vi "error_anal.vi"(9 "data":dbl[][](array[numeric])=array1024x498[509952 elements], 11 "wavelength":dbl[](array[numeric])=[350.0, 350.3, 350.6, 350.9, 351.2, 351.5, 351.8, 352.1, 352.4, 352.7, 353.0, 353.3, 353.6, 353.9, 354.2, 354.5, 354.8, 355.1, 355.4, 355.7, 356.0, 356.3, 356.6, 356.9, 357.2, 357.5, 357.8, 358.1, 358.4, 358.7, 359.0, 359.3, 359.6, 359.9, 360.2, 360.5, 360.8, 361.1, 361.4, 361.7, 362.0, 362.3, 362.6, 362.9, 363.2, 363.5, 363.8, 364.1, 364.4, 364.7, 365.0, 365.3, 365.6, 365.9, 366.2, 366.5, 366.8, 367.1, 367.4, 367.7, 368.0, 368.3, 368.6, 368.9, 369.2, 369.5, 369.8, 370.1, 370.4, 370.7, 371.0, 371.3, 371.6, 371.9, 372.2, 372.5, 372.8, 373.1, 373.4, 373.7, 374.0, 374.3, 374.6, 374.9, 375.2, 375.5, 375.8, 376.1, 376.4, 376.7, 377.0, 377.3, 377.6, 377.9, 378.2, 378.5, 378.8, 379.1, 379.4, 379.7, 380.0, 380.3, 380.6, 380.9, 381.2, 381.5, 381.8, 382.1, 382.4, 382.7, 383.0, 383.3, 383.6, 383.9, 384.2, 384.5, 384.8, 385.1, 385.4, 385.7, 386.0, 386.3, 386.6, 386.9, 387.2, 387.5, 387.8, 388.1, 388.4, 388.7, 389.0, 389.3, 389.6, 389.9, 390.2, 390.5, 390.8, 391.1, 391.4, 391.7, 392.0, 392.3, 392.6, 392.9, 393.2, 393.5, 393.8, 394.1, 394.4, 394.7, 395.0, 395.3, 395.6, 395.9, 396.2, 396.5, 396.8, 397.1, 397.4, 397.7, 398.0, 398.3, 398.6, 398.9, 399.2, 399.5, 399.8, 400.1, 400.4, 400.7, 401.0, 401.3, 401.6, 401.9, 402.2, 402.5, 402.8, 403.1, 403.4, 403.7, 404.0, 404.3, 404.6, 404.9, 405.2, 405.5, 405.8, 406.1, 406.4, 406.7, 407.0, 407.3, 407.6, 407.9, 408.2, 408.5, 408.8, 409.1, 409.4, 409.7, 410.0, 410.3, 410.6, 410.9, 411.2, 411.5, 411.8, 412.1, 412.4, 412.7, 413.0, 413.3, 413.6, 413.9, 414.2, 414.5, 414.8, 415.1, 415.4, 415.7, 416.0, 416.3, 416.6, 416.9, 417.2, 417.5, 417.8, 418.1, 418.4, 418.7, 419.0, 419.3, 419.6, 419.9, 420.2, 420.5, 420.8, 421.1, 421.4, 421.7, 422.0, 422.3, 422.6, 422.9, 423.2, 423.5, 423.8, 424.1, 424.4, 424.7, 425.0, 425.3, 425.6, 425.9, 426.2, 426.5, 426.8, 427.1, 427.4, 427.7, 428.0, 428.3, 428.6, 428.9, 429.2, 429.5, 429.8, 430.1, 430.4, 430.7, 431.0, 431.3, 431.6, 431.9, 432.2, 432.5, 432.8, 433.1, 433.4, 433.7, 434.0, 434.3, 434.6, 434.9, 435.2, 435.5, 435.8, 436.1, 436.4, 436.7, 437.0, 437.3, 437.6, 437.9, 438.2, 438.5, 438.8, 439.1, 439.4, 439.7, 440.0, 440.3, 440.6, 440.9, 441.2, 441.5, 441.8, 442.1, 442.4, 442.7, 443.0, 443.3, 443.6, 443.9, 444.2, 444.5, 444.8, 445.1, 445.4, 445.7, 446.0, 446.3, 446.6, 446.9, 447.2, 447.5, 447.8, 448.1, 448.4, 448.7, 449.0, 449.3, 449.6, 449.9, 450.2, 450.5, 450.8, 451.1, 451.4, 451.7, 452.0, 452.3, 452.6, 452.9, 453.2, 453.5, 453.8, 454.1, 454.4, 454.7, 455.0, 455.3, 455.6, 455.9, 456.2, 456.5, 456.8, 457.1, 457.4, 457.7, 458.0, 458.3, 458.6, 458.9, 459.2, 459.5, 459.8, 460.1, 460.4, 460.7, 461.0, 461.3, 461.6, 461.9, 462.2, 462.5, 462.8, 463.1, 463.4, 463.7, 464.0, 464.3, 464.6, 464.9, 465.2, 465.5, 465.8, 466.1, 466.4, 466.7, 467.0, 467.3, 467.6, 467.9, 468.2, 468.5, 468.8, 469.1, 469.4, 469.7, 470.0, 470.3, 470.6, 470.9, 471.2, 471.5, 471.8, 472.1, 472.4, 472.7, 473.0, 473.3, 473.6, 473.9, 474.2, 474.5, 474.8, 475.1, 475.4, 475.7, 476.0, 476.3, 476.6, 476.9, 477.2, 477.5, 477.8, 478.1, 478.4, 478.7, 479.0, 479.29999999999995, 479.6, 479.9, 480.2, 480.5, 480.79999999999995, 481.1, 481.4, 481.7, 482.0, 482.29999999999995, 482.6, 482.9, 483.2, 483.5, 483.79999999999995, 484.1, 484.4, 484.7, 485.0, 485.29999999999995, 485.6, 485.9, 486.2, 486.5, 486.79999999999995, 487.1, 487.4, 487.7, 488.0, 488.29999999999995, 488.6, 488.9, 489.2, 489.5, 489.79999999999995, 490.1, 490.4, 490.7, 491.0, 491.29999999999995, 491.6, 491.9, 492.2, 492.5, 492.79999999999995, 493.1, 493.4, 493.7, 494.0, 494.29999999999995, 494.6, 494.9, 495.2, 495.5, 495.79999999999995, 496.1, 496.4, 496.7, 497.0, 497.29999999999995, 497.6, 497.9, 498.2, 498.5, 498.79999999999995, 499.1, 499.4, 499.7, 500.0, 500.29999999999995, 500.6, 500.9, 501.2, 501.5, 501.79999999999995, 502.1, 502.4, 502.7, 503.0, 503.29999999999995, 503.6, 503.9, 504.2, 504.5, 504.79999999999995, 505.1, 505.4, 505.7, 506.0, 506.29999999999995, 506.6, 506.9, 507.2, 507.5, 507.79999999999995, 508.1, 508.4, 508.7, 509.0, 509.29999999999995, 509.6, 509.9, 510.2, 510.5, 510.79999999999995, 511.1, 511.4, 511.7, 512.0, 512.3, 512.6, 512.9, 513.2, 513.5, 513.8, 514.1, 514.4, 514.7, 515.0, 515.3, 515.6, 515.9, 516.2, 516.5, 516.8, 517.1, 517.4, 517.7, 518.0, 518.3, 518.6, 518.9, 519.2, 519.5, 519.8, 520.1, 520.4, 520.7, 521.0, 521.3, 521.6, 521.9, 522.2, 522.5, 522.8, 523.1, 523.4, 523.7, 524.0, 524.3, 524.6, 524.9, 525.2, 525.5, 525.8, 526.1, 526.4, 526.7, 527.0, 527.3, 527.6, 527.9, 528.2, 528.5, 528.8, 529.1, 529.4, 529.7, 530.0, 530.3, 530.6, 530.9, 531.2, 531.5, 531.8, 532.1, 532.4, 532.7, 533.0, 533.3, 533.6, 533.9, 534.2, 534.5, 534.8, 535.1, 535.4, 535.7, 536.0, 536.3, 536.6, 536.9, 537.2, 537.5, 537.8, 538.1, 538.4, 538.7, 539.0, 539.3, 539.6, 539.9, 540.2, 540.5, 540.8, 541.1, 541.4, 541.7, 542.0, 542.3, 542.6, 542.9, 543.2, 543.5, 543.8, 544.1, 544.4, 544.7, 545.0, 545.3, 545.6, 545.9, 546.2, 546.5, 546.8, 547.1, 547.4, 547.7, 548.0, 548.3, 548.6, 548.9, 549.2, 549.5, 549.8, 550.1, 550.4, 550.7, 551.0, 551.3, 551.6, 551.9, 552.2, 552.5, 552.8, 553.1, 553.4, 553.7, 554.0, 554.3, 554.6, 554.9, 555.2, 555.5, 555.8, 556.1, 556.4, 556.7, 557.0, 557.3, 557.6, 557.9, 558.2, 558.5, 558.8, 559.1, 559.4, 559.7, 560.0, 560.3, 560.6, 560.9, 561.2, 561.5, 561.8, 562.1, 562.4, 562.7, 563.0, 563.3, 563.6, 563.9, 564.2, 564.5, 564.8, 565.1, 565.4, 565.7, 566.0, 566.3, 566.6, 566.9, 567.2, 567.5, 567.8, 568.1, 568.4, 568.7, 569.0, 569.3, 569.6, 569.9, 570.2, 570.5, 570.8, 571.1, 571.4, 571.7, 572.0, 572.3, 572.6, 572.9, 573.2, 573.5, 573.8, 574.1, 574.4, 574.7, 575.0, 575.3, 575.6, 575.9, 576.2, 576.5, 576.8, 577.1, 577.4, 577.7, 578.0, 578.3, 578.6, 578.9, 579.2, 579.5, 579.8, 580.1, 580.4, 580.7, 581.0, 581.3, 581.6, 581.9, 582.2, 582.5, 582.8, 583.1, 583.4, 583.7, 584.0, 584.3, 584.6, 584.9, 585.2, 585.5, 585.8, 586.1, 586.4, 586.7, 587.0, 587.3, 587.6, 587.9, 588.2, 588.5, 588.8, 589.1, 589.4, 589.7, 590.0, 590.3, 590.6, 590.9, 591.2, 591.5, 591.8, 592.1, 592.4, 592.7, 593.0, 593.3, 593.6, 593.9, 594.2, 594.5, 594.8, 595.1, 595.4, 595.7, 596.0, 596.3, 596.6, 596.9, 597.2, 597.5, 597.8, 598.1, 598.4, 598.7, 599.0, 599.3, 599.6, 599.9, 600.2, 600.5, 600.8, 601.1, 601.4, 601.7, 602.0, 602.3, 602.6, 602.9, 603.2, 603.5, 603.8, 604.1, 604.4, 604.7, 605.0, 605.3, 605.6, 605.9, 606.2, 606.5, 606.8, 607.0999999999999, 607.4, 607.7, 608.0, 608.3, 608.5999999999999, 608.9, 609.2, 609.5, 609.8, 610.0999999999999, 610.4, 610.7, 611.0, 611.3, 611.5999999999999, 611.9, 612.2, 612.5, 612.8, 613.0999999999999, 613.4, 613.7, 614.0, 614.3, 614.5999999999999, 614.9, 615.2, 615.5, 615.8, 616.0999999999999, 616.4, 616.7, 617.0, 617.3, 617.5999999999999, 617.9, 618.2, 618.5, 618.8, 619.0999999999999, 619.4, 619.7, 620.0, 620.3, 620.5999999999999, 620.9, 621.2, 621.5, 621.8, 622.0999999999999, 622.4, 622.7, 623.0, 623.3, 623.5999999999999, 623.9, 624.2, 624.5, 624.8, 625.0999999999999, 625.4, 625.7, 626.0, 626.3, 626.5999999999999, 626.9, 627.2, 627.5, 627.8, 628.0999999999999, 628.4, 628.7, 629.0, 629.3, 629.5999999999999, 629.9, 630.2, 630.5, 630.8, 631.0999999999999, 631.4, 631.7, 632.0, 632.3, 632.5999999999999, 632.9, 633.2, 633.5, 633.8, 634.0999999999999, 634.4, 634.7, 635.0, 635.3, 635.5999999999999, 635.9, 636.2, 636.5, 636.8, 637.0999999999999, 637.4, 637.7, 638.0, 638.3, 638.5999999999999, 638.9, 639.2, 639.5, 639.8, 640.0999999999999, 640.4, 640.7, 641.0, 641.3, 641.5999999999999, 641.9, 642.2, 642.5, 642.8, 643.0999999999999, 643.4, 643.7, 644.0, 644.3, 644.5999999999999, 644.9, 645.2, 645.5, 645.8, 646.0999999999999, 646.4, 646.7, 647.0, 647.3, 647.5999999999999, 647.9, 648.2, 648.5, 648.8, 649.0999999999999, 649.4, 649.7, 650.0, 650.3, 650.5999999999999, 650.9, 651.2, 651.5, 651.8, 652.0999999999999, 652.4, 652.7, 653.0, 653.3, 653.5999999999999, 653.9, 654.2, 654.5, 654.8, 655.0999999999999, 655.4, 655.7, 656.0, 656.3, 656.5999999999999, 656.9]) -> ()   [LabVIEW 2019]
uses:
  <vilib>/Analysis/NI_AALBase.lvlib
panel:
  out "error anal 6":T1(graph)={"Histogram: h(x)"=[4, 2, 9, 18, 33, 50, 62, 78, 72, 64, 50, 29, 23, 2, 2], "X Values"=[-207.47593984155532, -179.342606508222, -151.20927317488866, -123.07593984155534, -94.94260650822201, -66.80927317488869, -38.675939841555355, -10.542606508222022, 17.59072682511131, 45.724060158444644, 73.85739349177797, 101.9907268251113, 130.12406015844462, 158.25739349177795, 186.39072682511127]}
  out "error anal 5":T1(graph)={"Histogram: h(x)"=[4, 11, 26, 31, 53, 82, 83, 67, 59, 46, 18, 11, 6, 0, 1], "X Values"=[-169.02894487542682, -141.13697283069715, -113.24500078596748, -85.35302874123781, -57.461056696508145, -29.569084651778482, -1.6771126070488194, 26.214859437680843, 54.106831482410506, 81.99880352714017, 109.89077557186982, 137.7827476165995, 165.67471966132916, 193.56669170605883, 221.4586637507885]}
  out "error anal 4":T1(graph)={"Histogram: h(x)"=[2, 5, 14, 39, 67, 69, 32, 22, 21, 29, 50, 68, 49, 21, 10], "X Values"=[-360.2067266548067, -312.64850810225613, -265.0902895497056, -217.53207099715505, -169.97385244460452, -122.41563389205399, -74.85741533950346, -27.299196786952926, 20.25902176559761, 67.81724031814815, 115.37545887069868, 162.9336774232492, 210.49189597579974, 258.05011452835026, 305.6083330809008]}
  out "error anal 3":cluster{i32[], dbl[]}(graph)
  out "error anal 2":cluster{i32[], dbl[]}(graph)
  out "error anal 2":cluster{i32[], dbl[]}(graph)
  out "error anal":cluster{"wavelength":dbl[], dbl[]}[](graph)
  out "camera":cluster{"wavelength":dbl[], dbl[]}[](graph)
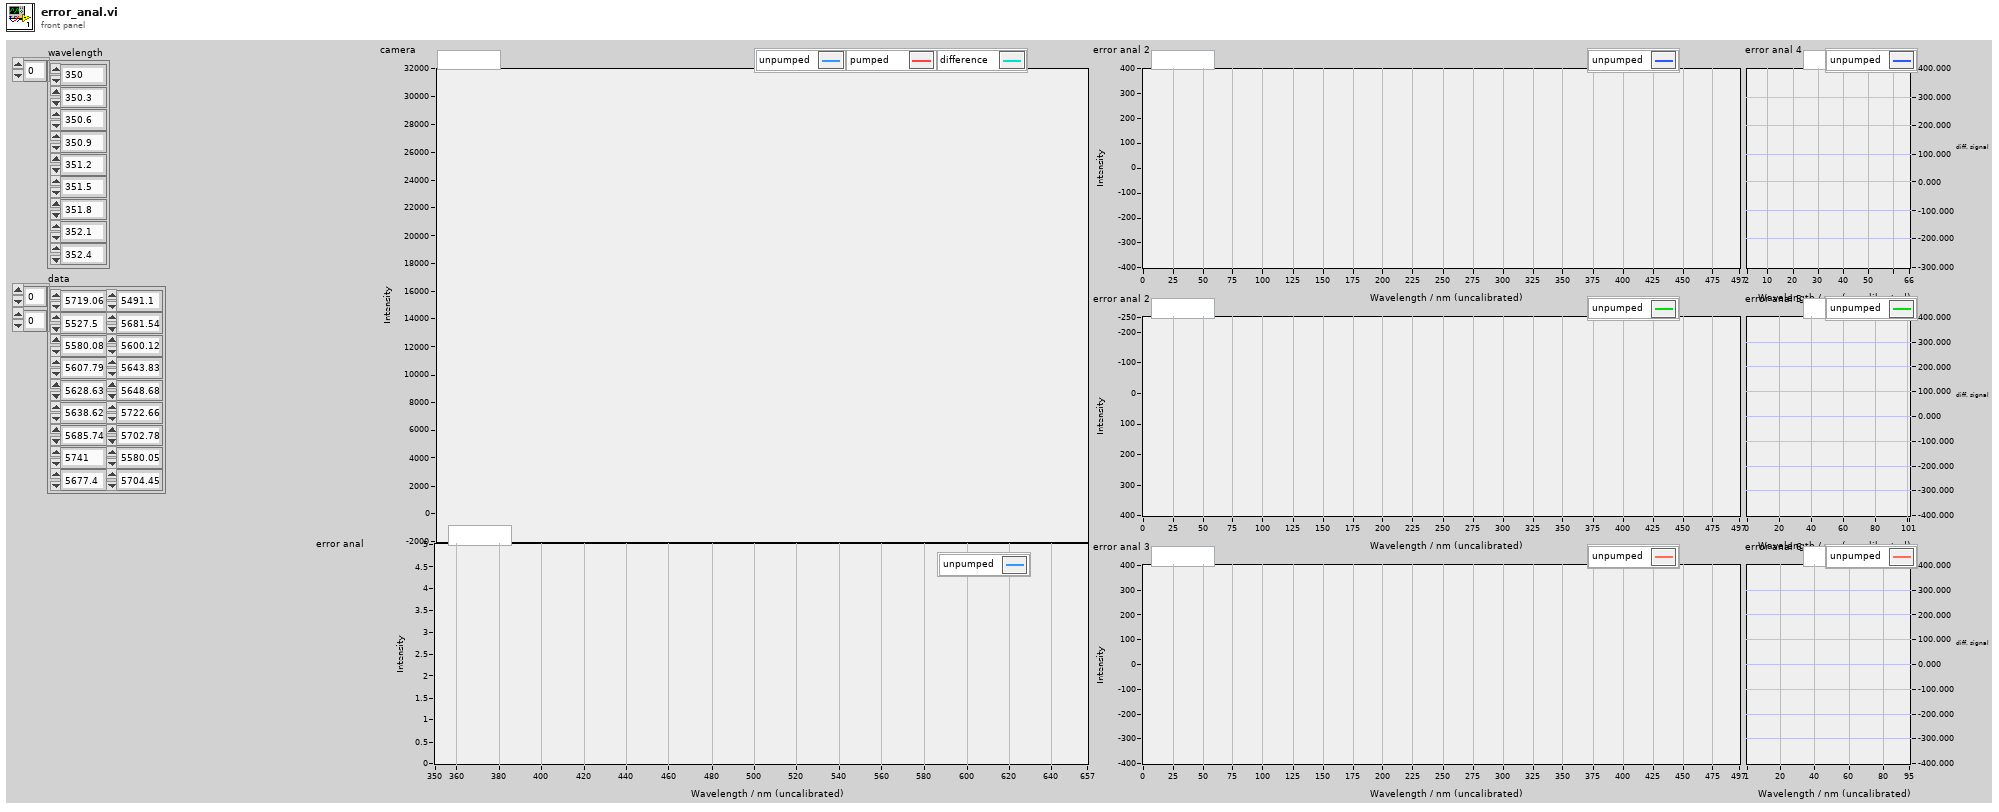
[diagram p1: front panel]
types:
  T1 = cluster{"Histogram: h(x)":i32[], "X Values":dbl[]}
  T2 = enum32{"Invalid", "Standard", "Closed", "Hidden", "Minimized", "Maximized"}
  T3 = typedef "LVCursorListTypeDef.ctl" = cluster{"Name":string, "Color":u32, "Style":u8, "Point Style":u8, "Name Visible":bool, "Allow Drag":bool, "Cursor Mode":u32, "Plot":i32, "Index":i32, "Position":cluster{"X":dbl, "Y":dbl}, "X Scale":u32, "Y Scale":u32, "Watch Plots":i32[], "Watch All Plots":bool, "Plot Area":i32, "Label Offset":cluster{"X":dbl, "Y":dbl}}[]
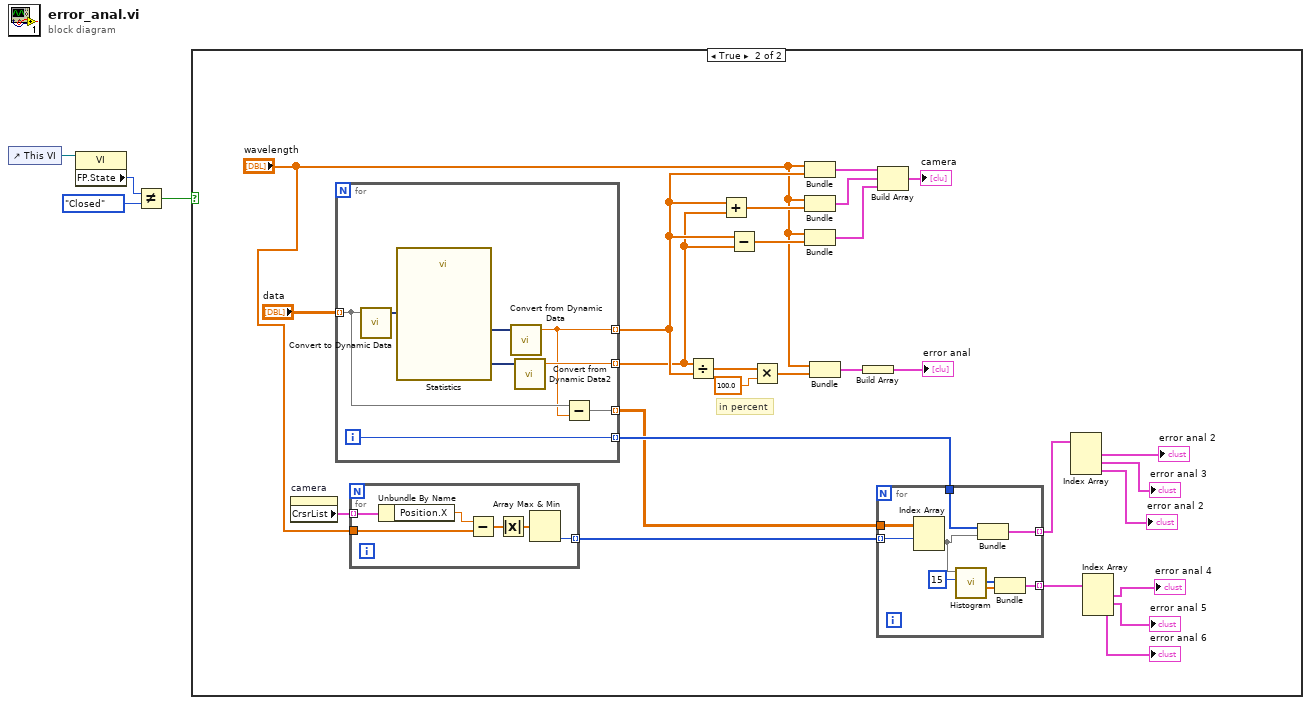
[diagram p0: block diagram]
diagram:
  n1 = control-ref of="This VI"() -> (w4:refnum<vi>)
  n2 = property class="VI"(reference=w4) -> ("FP.State"=w3:T2)  [unwired: 1 in, 2 out]
  n3 = Not Equal?(x=w3, y=T2."Closed") -> (x != y?=w1:bool)
  n4 = case shown="True" w1 {
    frame False {
    }
    frame True {
      # "in percent"
      n5 = property on="camera" class="XYGraph (strict)"() -> ("CrsrList"=w16:T3)  [unwired: 2 in, 2 out]
      n6 = for {
        tunnel: "data" -> [w49] mode=indexing
        tunnel: [w48] -> w25 mode=indexing
        tunnel: [w52] -> w24 mode=indexing
        tunnel: [w50] -> w18 mode=indexing
        tunnel: [w47] -> w13 mode=indexing
        i -> [w50]
        n7 = call "Convert to Dynamic Data"("Array"=w49) -> ("Dynamic Data Type"=w54:dynamicdata)  [unwired: 3 in]
        n8 = call "Statistics"("Signals"=w54) -> ("Standard Dev"=w51:dynamicdata, "Arithmetic Mean"=w53:dynamicdata)  [unwired: 23 in, 2 out]
        n9 = call "Convert from Dynamic Data"("Dynamic Data Type"=w53) -> ("Scalar"=w48:dbl)  [unwired: 3 in]
        n10 = call "Convert from Dynamic Data2"("Dynamic Data Type"=w51) -> ("Scalar"=w52:dbl)  [unwired: 3 in]
        n11 = Subtract(x=w49, y=w48) -> (x-y=w47:dbl[])
      }
      n12 = for {
        tunnel: w16 -> [w46] mode=indexing
        tunnel: [w41] -> w14 mode=indexing
        tunnel: "wavelength" -> [w44]
        n13 = Unbundle By Name(w46) -> ("Position.X"=w45:dbl)
        n14 = Subtract(x=w45, y=w44) -> (x-y=w43:dbl[])
        n15 = Absolute Value(x=w43) -> (abs(x)=w42:dbl[])
        n16 = Array Max & Min(array=w42) -> (min index (indices)=w41:i32)  [unwired: 3 out]
      }
      n17 = Divide(x=w24, y=w25) -> (x/y=w31:dbl[])
      n18 = Add(x=w25, y=w24) -> (x+y=w27:dbl[])
      n19 = Subtract(x=w25, y=w24) -> (x-y=w23:dbl[])
      n20 = Multiply(x=w31, y=100.0) -> (x*y=w30:dbl[])
      n21 = Bundle("wavelength"="wavelength", w25) -> (w29:cluster{"wavelength":dbl[], dbl[]})  [unwired: 1 in]
      n22 = Bundle("wavelength"="wavelength", w27) -> (w26:cluster{"wavelength":dbl[], dbl[]})  [unwired: 1 in]
      n23 = Bundle("wavelength"="wavelength", w23) -> (w22:cluster{"wavelength":dbl[], dbl[]})  [unwired: 1 in]
      n24 = Bundle("wavelength"="wavelength", w30) -> (w21:cluster{"wavelength":dbl[], dbl[]})  [unwired: 1 in]
      n25 = Build Array(w21) -> (→"error anal":cluster{"wavelength":dbl[], dbl[]}[])
      n26 = for {
        tunnel: w13 -> [w40]
        tunnel: [w39] -> w12 mode=indexing
        tunnel: w18 -> [w38]
        tunnel: w14 -> [w37] mode=indexing
        tunnel: [w33] -> w8 mode=indexing
        n27 = Index Array(array=w40, index (row)=w37) -> (element=w36:dbl[])  [unwired: 1 in]
        n28 = call <vilib>:"Histogram.vi"("intervals"=15, "X"=w36) -> ("X Values"=w35:dbl[], "Histogram: h(x)"=w34:i32[])  [unwired: 6 in, 2 out]
        n29 = Bundle(w38, w36) -> (w39:cluster{i32[], dbl[]})  [unwired: 1 in]
        n30 = Bundle("Histogram: h(x)"=w34, "X Values"=w35) -> (w33:T1)  [unwired: 1 in]
      }
      n31 = Build Array(w29, w26, w22) -> (→"camera":cluster{"wavelength":dbl[], dbl[]}[])
      n32 = Index Array(array=w12) -> (element #1=→"error anal 2":cluster{i32[], dbl[]}, element #2=→"error anal 3":cluster{i32[], dbl[]}, element #3=→"error anal 2":cluster{i32[], dbl[]})  [unwired: 3 in]
      n33 = Index Array(array=w8) -> (element #1=→"error anal 4":T1, element #2=→"error anal 5":T1, element #3=→"error anal 6":T1)  [unwired: 3 in]
    }
  }
